vi "Test Lockin API.vi"() -> ()   [LabVIEW 2016]
uses:
  src/Instrument.Lockin/Instrument.Lockin.lvclass
  <vilib>/addons/_JKI Toolkits/Caraya/classes/Test Suite/Define Test Suite (Default).vi
  <vilib>/addons/_JKI Toolkits/Caraya/classes/Test Suite/Test Suite.lvclass
panel:
  out "Instrument.Lockin out":refnum<class "Instrument.Lockin.lvclass">
  in  "Instrument.Lockin in":refnum<class "Instrument.Lockin.lvclass">
  # "TEST"
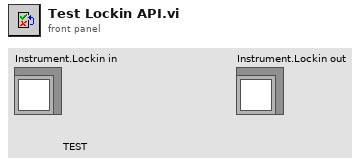
[diagram p1: front panel]
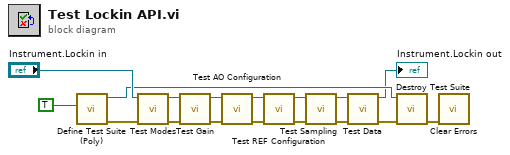
[diagram p0: block diagram]
diagram:
  n1 = call-poly <vilib>:"Define Test Suite (Poly).vi"("Interactive"=TRUE) -> ("error out"=w12:errorcluster, "Test Suite"=w10:refnum<class "Test Suite.lvclass">)  [unwired: 9 in]
  n2 = call "Test Modes.vi"("error in (no error)"=w12, "Instrument.Lockin in"="Instrument.Lockin in") -> ("error out"=w8:errorcluster, "Instrument.Lockin out"=w17:refnum<class "Instrument.Lockin.lvclass">)  [unwired: 8 in]
  n3 = call "Test Gain.vi"("error in (no error)"=w8, "Instrument.Lockin in"=w17) -> ("error out"=w7:errorcluster, "Instrument.Lockin out"=w16:refnum<class "Instrument.Lockin.lvclass">)  [unwired: 8 in]
  n4 = call "Test AO Configuration.vi"("error in (no error)"=w7, "Instrument.Lockin in"=w16) -> ("error out"=w6:errorcluster, "Instrument.Lockin out"=w15:refnum<class "Instrument.Lockin.lvclass">)  [unwired: 8 in]
  n5 = call "Test REF Configuration.vi"("error in (no error)"=w6, "Instrument.Lockin in"=w15) -> ("error out"=w5:errorcluster, "Instrument.Lockin out"=w14:refnum<class "Instrument.Lockin.lvclass">)  [unwired: 8 in]
  n6 = call "Test Sampling.vi"("error in (no error)"=w5, "Instrument.Lockin in"=w14) -> ("error out"=w4:errorcluster, "Instrument.Lockin out"=w13:refnum<class "Instrument.Lockin.lvclass">)  [unwired: 8 in]
  n7 = call "Test Data.vi"("error in (no error)"=w4, "Instrument.Lockin in"=w13) -> ("error out"=w3:errorcluster, "Instrument.Lockin out"=→"Instrument.Lockin out":refnum<class "Instrument.Lockin.lvclass">)  [unwired: 8 in]
  n8 = call-dynamic "Destroy Test Suite.vi"("error in (no error)"=w3, "Test Suite in"=w10) -> ("error out"=w1:errorcluster)  [unwired: 9 in]
  n9 = call <vilib>:"Clear Errors.vi"("error in (no error)"=w1) -> ()  [unwired: 5 in, 2 out]
